vi "sv_Convert Spectrum Info to Variant Attributes.vi"(6 "LabVIEW datatype":T6=3 items=["String: abc"=7, "Boolean: True or False"=8, "Scalar: y"=0, "Array: Y"=1, "Waveform: t0, dt, Y, variant"=2, "Cluster: x0, dx, Y"=3, "Cluster: X, Y"=4, "Waterfall"=5, "Colormap"=6], 8 "error in":errorcluster, 9 "spectrum info":T8 {"x-axis units" items=["Time (s)"=0, "Frequency-CB (Hz)"=1, "Frequency-CPB (Hz)"=1248, "Frequency-Arbitrary (Hz)"=2357, "Quefrency (s)"=2, "Revolutions (rev)"=3, "Order"=4, "Speed (RPM)"=11, "Speed (rad/s)"=21, "Index"=65535]; "weighting filter" items=["Linear", "A-weighting", "B-weighting", "C-weighting", "ITU-R 468-4", "Dolby", "CCITT", "C-message", "Wb", "Wc", "Wd", "We", "Wf", "Wh", "Wj", "Wk", "Wm", "AES17 20 kHz lowpass", "AES17 40 kHz lowpass", "AES17 20 kHz highpass", "AES17 40 kHz highpass"]; "dB reference [EU]" format="%.2f"; "engineering units" items=["custom..."=0, "V"=1, "A"=21, "C"=30, "pC"=31, "s"=32, "-"=29, "Pa"=2, "N"=20, "g"=3, "m/s^2"=4, "m/s"=5, "m"=6, "mm/s"=12, "mm"=13, "micron/s"=14, "micron"=15, "in/s^2"=7, "in/s"=8, "in"=9, "mil/s"=10, "mil"=11, "rad/s^2"=16, "rad/s"=17, "rad"=18, "deg/s^2"=26, "deg/s"=27, "deg"=28, "RPM"=22, "cycle/s^2"=23, "Hz"=24, "cycle"=25, "strain"=19]; "spectral info"."window" items=["None "=0, "Hanning"=1, "Hamming"=2, "Blackman-Harris"=3, "Exact Blackman"=4, "Blackman"=5, "Flat Top"=6, "4 Term B-Harris "=7, "7 Term B-Harris"=8, "Low Sidelobe"=9, "Force - Exponential"=10, "Gaussian"=62]}, 10 "spectrum component":T7 items=["Magnitude"=32, "Phase"=33, "Real"=34, "Imaginary"=35, "Coherence"=36, "Unknown"=99], 11 "attributes in":variant) -> (0 "error out":errorcluster, 1 "unit info":T5, 2 "function info":T4 {"function type" items=["Signal"=0, "Speed"=3, "Ratio"=6, "Count"=7, "-"=9, "Level"=10, "-"=19, "Octave Spectrum"=20, "-"=29, "FFT Auto Spectrum"=30, "FFT Cross Spectrum"=40, "Frequency Response"=50, "-"=59, "Event"=90]; "function subtype" items=["Unscaled binary"=0, "Scaled voltage"=1, "Scaled engineering units"=2, "-"=10, "Value"=19, "DC"=11, "AC"=12, "RMS^2"=13, "RMS"=14, "Peak"=15, "Peak to peak"=16, "-"=20, "1/1 octave"=21, "1/3 octave"=22, "1/6 octave"=23, "1/12 octave"=24, "1/24 octave"=25, "-"=30, "Density"=31, "Magnitude"=32, "Phase"=33, "Real"=34, "Imaginary"=35, "Complex"=345, "Coherence"=36, "-"=90, "Unknown"=99]; "X-domain" items=["Time (s)"=0, "Frequency-CB (Hz)"=1, "Frequency-CPB (Hz)"=1248, "Frequency-Arbitrary (Hz)"=2357, "Quefrency (s)"=2, "Revolutions (rev)"=3, "Order"=4, "Speed (RPM)"=11, "Speed (rad/s)"=21, "Index"=65535]}, 3 "attributes out":variant)   [LabVIEW 2017]
uses:
  <vilib>/addons/_NISVFA/_Shared subVIs/Controls/svc_Spectrum Info.ctl
  <vilib>/addons/_NISVFA/_Shared subVIs/Controls/svc_X-Axis Units.ctl
  <vilib>/addons/_NISVFA/_Shared subVIs/Controls/svc_Spectrum Type.ctl
  <vilib>/addons/_NISVFA/_Shared subVIs/Controls/svc_Engineering Units Text Ring.ctl
  <vilib>/addons/_NISVFA/_Shared subVIs/Controls/svc_Weighting Filter Text Ring.ctl
  <vilib>/addons/_NISVFA/_Shared subVIs/Controls/svc_Complimentary Spectrum Units.ctl
  <vilib>/addons/_NISVFA/_Shared subVIs/Controls/NI Spectrum Component.ctl
  <vilib>/addons/_NISVFA/_Shared subVIs/Controls/LV Datatypes.ctl
  <vilib>/addons/_NISVFA/_Shared subVIs/Controls/NI Function Type.ctl
  <vilib>/addons/_NISVFA/_Shared subVIs/Controls/NI Function SubType.ctl
  <vilib>/addons/_NISVFA/_Shared subVIs/Controls/NI Channel Properties.ctl
  <vilib>/addons/_NISVFA/_Shared subVIs/Controls/SV Channel Properties.ctl
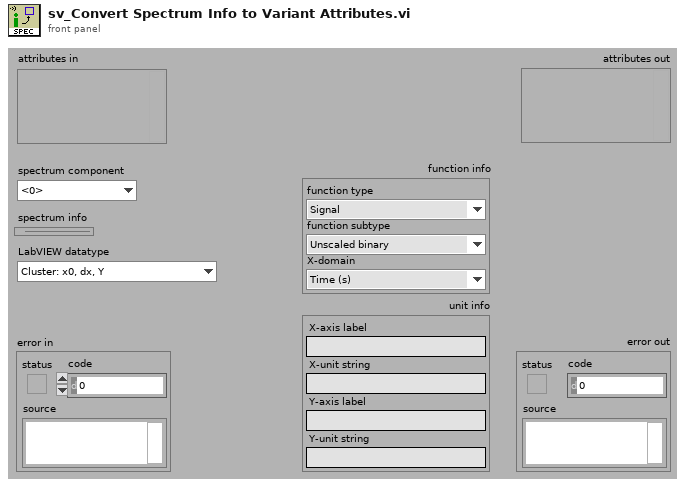
[diagram p1: front panel]
types:
  T1 = typedef "NI Function Type.ctl" = u16
  T2 = typedef "NI Function SubType.ctl" = u16
  T3 = typedef "svc_X-Axis Units.ctl" = u16
  T4 = cluster{"function type":T1, "function subtype":T2, "X-domain":T3}
  T5 = cluster{"X-axis label":string, "X-unit string":string, "Y-axis label":string, "Y-unit string":string}
  T6 = typedef "LV Datatypes.ctl" = i32
  T7 = typedef "NI Spectrum Component.ctl" = u16
  T8 = typedef "svc_Spectrum Info.ctl" = cluster{"channel name":string, "description":string, "x-axis units":T3, "spectral info":cluster{"spectrum type":T9, "linear/dB":enum16{"linear", "dB"}, "window":u16, "window size":i32, "FFT size":i32}, "engineering units":T10, "custom label":string, "dB reference [EU]":dbl, "peak units":enum16{"rms", "peak", "peak-peak"}, "weighting filter":T11, "spectral density?":bool, "unit label":string, "spectrum skewed?":bool, "complimentary spectrum units":T12}
  T9 = typedef "svc_Spectrum Type.ctl" = enum16{"FFT Spectrum [complex]", "Amplitude [Magnitude]", "Power [Magnitude^2]", "Cross Spectrum [complex]", "Frequency Response [Complex]"}
  T10 = typedef "svc_Engineering Units Text Ring.ctl" = u16
  T11 = typedef "svc_Weighting Filter Text Ring.ctl" = u16
  T12 = typedef "svc_Complimentary Spectrum Units.ctl" = enum16{"none", "radians", "degrees", "cycles", "imaginary"}
  T13 = typedef "NI Channel Properties.ctl" = u16
  T14 = typedef "SV Channel Properties.ctl" = u16
  T15 = enum16{"No averaging", "Vector averaging", "RMS averaging", "Peak hold"}
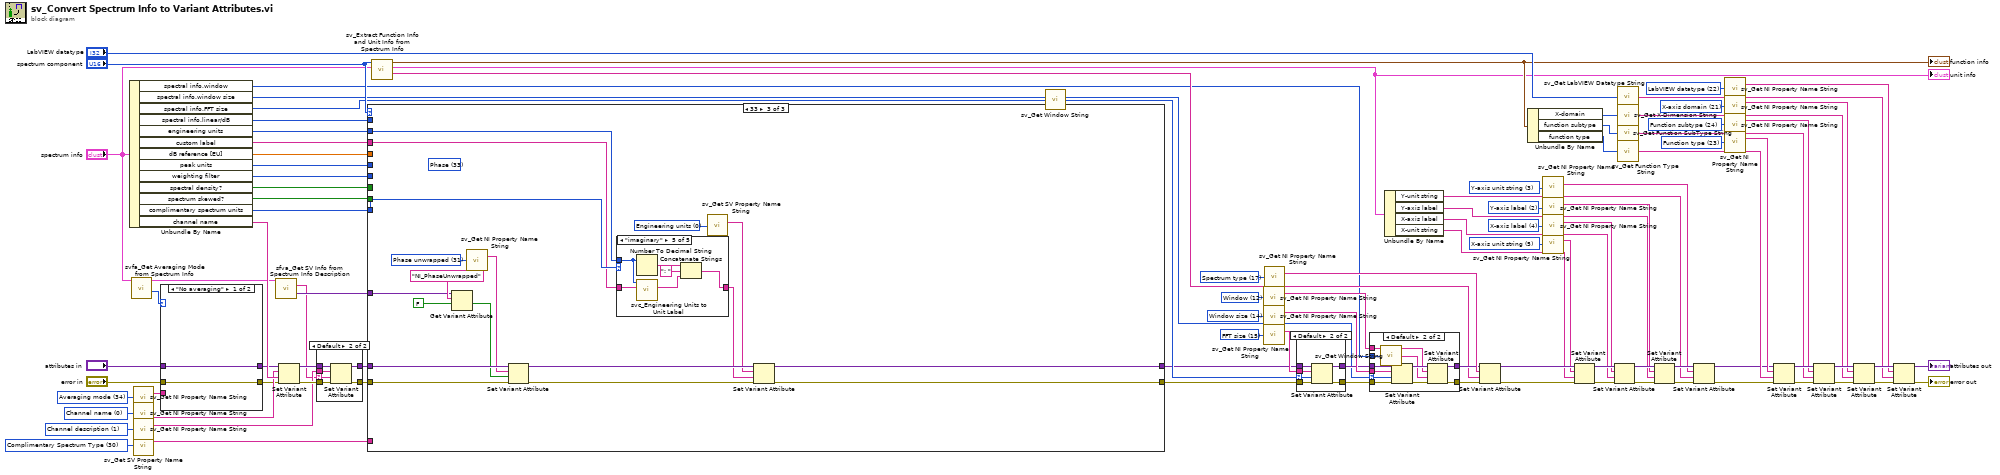
[diagram p0: block diagram]
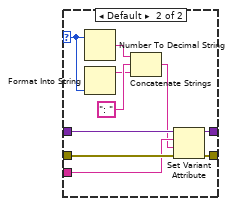
[diagram p2: hidden frame]
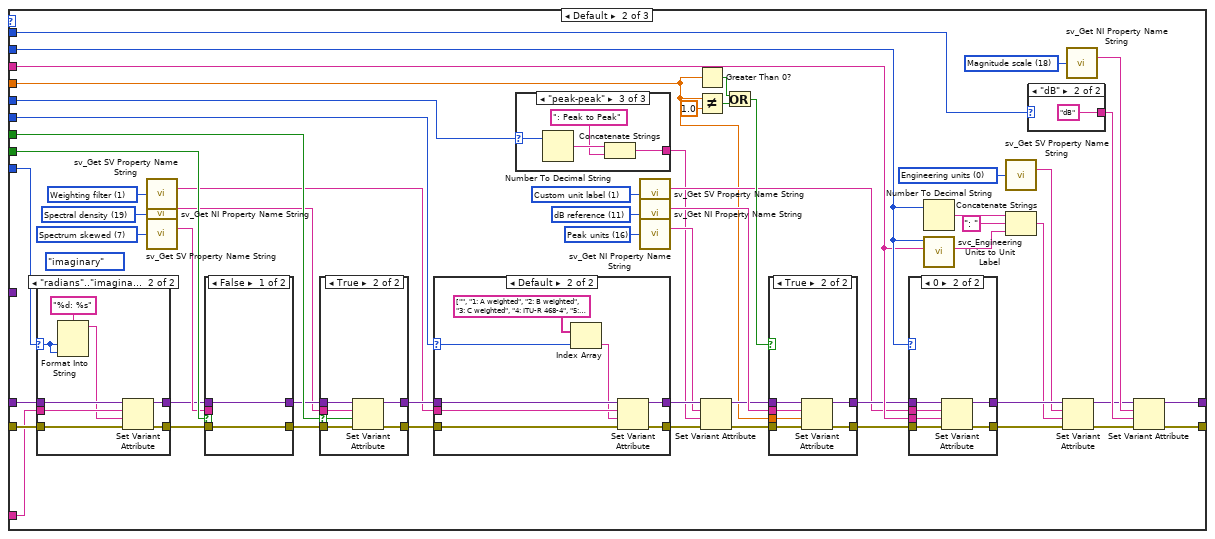
[diagram p7: hidden frame]
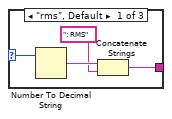
[diagram p10: hidden frame]
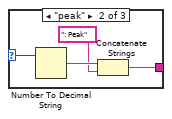
[diagram p11: hidden frame]
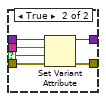
[diagram p12: hidden frame]
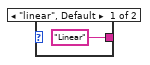
[diagram p13: hidden frame]
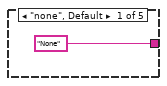
[diagram p17: hidden frame]
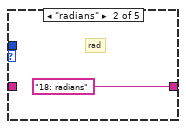
[diagram p18: hidden frame]
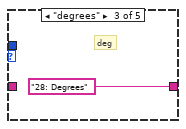
[diagram p19: hidden frame]
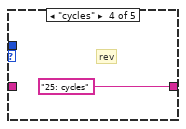
[diagram p20: hidden frame]
diagram:
  w3 = T13 34 items=["Channel name", "Channel description", "Axis label", "Unit string", "Waveform X-axis label", "Waveform X-axis unit string", "x0", "dx", "Number of samples", "X channel", "Filter settled", "dB reference", "Window", "Window parameter", "Window size", "FFT size", "Peak units", "Spectrum type", "Magnitude scale", "Spectral density", "Sensor sensitivity (mV/EU)", "X-axis dimension", "LabVIEW datatype", "Function type", "Function subtype", "X values", "Independent channel", "Column index", "Collection name", "Collection ID", "X Columns", "Phase unwrapped", "Sensor type", "Sensor maximum", "Averaging mode"] ("property")
  w12 = T14 30 items=["Engineering units", "Custom unit label", "Weighting filter", "Pregain", "Octave standard", "Octave bandwidth", "Octave low band", "Octave high band", "Spectrum skewed", "Samples / revolution", "Order", "Tachometer", "Pulses Per Revolution", "Rotation Direction", "Probe Angle", "Pair", "Channel Alias", "Tachometer Threshold", "Tachometer Slope", "Max Order", "Sensor Location", "Sensor Orientation", "Analog Software Trigger", "Trigger Level", "Pretrigger Samples", "Trigger Slope", "Trigger Hysteresis", "Sensor sensitivity", "Sensor type", "Sensor maximum", "Complimentary Spectrum Type"] ("property")
  w33 = T13 2 items=["Channel name", "Channel description", "Y-axis label", "Y-axis unit string", "X-axis label", "X-axis unit string", "x0", "dx", "Number of samples", "X channel", "Filter settled", "dB reference", "Window", "Window parameter", "Window size", "FFT size", "Peak units", "Spectrum type", "Magnitude scale", "Spectral density", "Sensor sensitivity (mV/EU)", "X-axis domain", "LabVIEW datatype"] ("property")
  w32 = T13 3 items=["Channel name", "Channel description", "Y-axis label", "Y-axis unit string", "X-axis label", "X-axis unit string", "x0", "dx", "Number of samples", "X channel", "Filter settled", "dB reference", "Window", "Window parameter", "Window size", "FFT size", "Peak units", "Spectrum type", "Magnitude scale", "Spectral density", "Sensor sensitivity (mV/EU)", "X-axis domain", "LabVIEW datatype"] ("property")
  w35 = T13 5 items=["Channel name", "Channel description", "Y-axis label", "Y-axis unit string", "X-axis label", "X-axis unit string", "x0", "dx", "Number of samples", "X channel", "Filter settled", "dB reference", "Window", "Window parameter", "Window size", "FFT size", "Peak units", "Spectrum type", "Magnitude scale", "Spectral density", "Sensor sensitivity (mV/EU)", "X-axis domain", "LabVIEW datatype"] ("property")
  w36 = T13 4 items=["Channel name", "Channel description", "Y-axis label", "Y-axis unit string", "X-axis label", "X-axis unit string", "x0", "dx", "Number of samples", "X channel", "Filter settled", "dB reference", "Window", "Window parameter", "Window size", "FFT size", "Peak units", "Spectrum type", "Magnitude scale", "Spectral density", "Sensor sensitivity (mV/EU)", "X-axis domain", "LabVIEW datatype"] ("property")
  w49 = T13 15 items=["Channel name", "Channel description", "Y-axis label", "Y-axis unit string", "X-axis label", "X-axis unit string", "x0", "dx", "Number of samples", "X channel", "Filter settled", "dB reference", "Window", "Window parameter", "Window size", "FFT size", "Peak units", "Spectrum type", "Magnitude scale", "Spectral density"] ("property")
  w48 = T13 14 items=["Channel name", "Channel description", "Y-axis label", "Y-axis unit string", "X-axis label", "X-axis unit string", "x0", "dx", "Number of samples", "X channel", "Filter settled", "dB reference", "Window", "Window parameter", "Window size", "FFT size", "Peak units", "Spectrum type", "Magnitude scale", "Spectral density"] ("property")
  w45 = T13 12 items=["Channel name", "Channel description", "Y-axis label", "Y-axis unit string", "X-axis label", "X-axis unit string", "x0", "dx", "Number of samples", "X channel", "Filter settled", "dB reference", "Window", "Window parameter", "Window size", "FFT size", "Peak units", "Spectrum type", "Magnitude scale", "Spectral density"] ("property")
  w70 = T13 22 items=["Channel name", "Channel description", "Y-axis label", "Y-axis unit string", "X-axis label", "X-axis unit string", "x0", "dx", "Number of samples", "X channel", "Filter settled", "dB reference", "Window", "Window parameter", "Window size", "FFT size", "Peak units", "Spectrum type", "Magnitude scale", "Spectral density", "Sensor sensitivity (mV/EU)", "X-axis domain", "LabVIEW datatype"] ("property")
  w73 = T13 24 items=["Channel name", "Channel description", "Y-axis label", "Y-axis unit string", "X-axis label", "X-axis unit string", "x0", "dx", "Number of samples", "X channel", "Filter settled", "dB reference", "Window", "Window parameter", "Window size", "FFT size", "Peak units", "Spectrum type", "Magnitude scale", "Spectral density", "Sensor sensitivity (mV/EU)", "X-axis dimension", "LabVIEW datatype", "Function type", "Function subtype"] ("property")
  w74 = T13 21 items=["Channel name", "Channel description", "Y-axis label", "Y-axis unit string", "X-axis label", "X-axis unit string", "x0", "dx", "Number of samples", "X channel", "Filter settled", "dB reference", "Window", "Window parameter", "Window size", "FFT size", "Peak units", "Spectrum type", "Magnitude scale", "Spectral density", "Sensor sensitivity (mV/EU)", "X-axis domain", "LabVIEW datatype", "Function type", "Component", "Level detector"] ("property")
  w72 = T13 23 items=["Channel name", "Channel description", "Y-axis label", "Y-axis unit string", "X-axis label", "X-axis unit string", "x0", "dx", "Number of samples", "X channel", "Filter settled", "dB reference", "Window", "Window parameter", "Window size", "FFT size", "Peak units", "Spectrum type", "Magnitude scale", "Spectral density", "Sensor sensitivity (mV/EU)", "X-axis domain", "LabVIEW datatype", "Function type", "Component", "Level detector"] ("property")
  w93 = T13 17 items=["Channel name", "Channel description", "Y-axis label", "Y-axis unit string", "X-axis label", "X-axis unit string", "x0", "dx", "Number of samples", "X channel", "Filter settled", "dB reference", "Window", "Window parameter", "Window size", "FFT size", "Peak units", "Spectrum type", "Magnitude scale", "Spectral density"] ("property")
  w92 = T13 0 items=["Channel name", "Channel description", "Y-axis label", "Y-axis unit string", "X-axis label", "X-axis unit string", "x0", "dx", "Number of samples", "X channel", "Filter settled", "dB reference", "Window", "Window parameter", "Window size", "FFT size", "Peak units", "Spectrum type", "Magnitude scale", "Spectral density"] ("property")
  w91 = T13 1 items=["Channel name", "Channel description", "Y-axis label", "Y-axis unit string", "X-axis label", "X-axis unit string", "x0", "dx", "Number of samples", "X channel", "Filter settled", "dB reference", "Window", "Window parameter", "Window size", "FFT size", "Peak units", "Spectrum type", "Magnitude scale", "Spectral density"] ("property")
  n1 = Unbundle By Name("spectrum info") -> ("spectral info.window"=w13:u16, "spectral info.window size"=w39:i32, "spectral info.FFT size"=w44:i32, "spectral info.linear/dB"=w84:enum16{"linear", "dB"}, "engineering units"=w85:T10, "custom label"=w86:string, "dB reference [EU]"=w87:dbl, "peak units"=w90:enum16{"rms", "peak", "peak-peak"}, "weighting filter"=w88:T11, "spectral density?"=w95:bool, "spectrum skewed?"=w83:bool, "complimentary spectrum units"=w89:T12, "channel name"=w37:string)
  n2 = call <vilib>:"svfa_Get Averaging Mode from Spectrum Info.vi"("spectrum info"="spectrum info") -> ("averaging mode"=w1:T15, "spectrum info"=w8:T8)  [unwired: 8 in, 1 out]
  n3 = call <vilib>:"sv_Get NI Property Name String.vi"("property"=w3) -> ("TDMS property name"=w2:string)  [unwired: 13 in, 1 out]
  n4 = call <vilib>:"sv_Get NI Property Name String.vi"("property"=w92) -> ("WDT attribute name"=w10:string)  [unwired: 13 in, 1 out]
  n5 = call <vilib>:"sv_Get NI Property Name String.vi"("property"=w91) -> ("TDMS property name"=w80:string)  [unwired: 13 in, 1 out]
  n6 = call <vilib>:"sv_Get SV Property Name String.vi"("property"=w12) -> ("TDMS property name"=w11:string)  [unwired: 13 in, 1 out]
  n7 = case shown="\"No averaging\"" w1 {
    selector: w1 -> [_ w102]
    tunnel: "attributes in" -> [w100 w110]
    tunnel: [w100 w109] -> w6
    tunnel: "error in" -> [w99 w108]
    tunnel: [w99 w107] -> w4
    tunnel: w2 -> [_ w106]
    frame "No averaging" {
    }
    frame Default {
      n8 = Number To Decimal String(number=w102) -> (decimal integer string=w104:string)  [unwired: 1 in]
      n9 = Format Into String(w102) -> (resulting string=w103:string)  [unwired: 3 in, 1 out]
      n10 = Concatenate Strings(w104, ": " ("string"), w103) -> (w101:string)
      n11 = Set Variant Attribute(Variant=w110, name=w106, value=w101, error in=w108) -> (Variant out=w109:variant, error out=w107:errorcluster)  [unwired: 1 out]
    }
  }
  n12 = call <vilib>:"sfva_Get SV Info from Spectrum Info Description.vi"("spectrum info"=w8) -> ("description"=w79:string, "SV Info"=w98:variant)  [unwired: 10 in, 3 out]
  n13 = Set Variant Attribute(Variant=w6, name=w10, value=w37, error in=w4) -> (Variant out=w82:variant, error out=w81:errorcluster)  [unwired: 1 out]
  n14 = case shown="Default" w79 {
    selector: w79 -> [_ w114]
    tunnel: [w112 w115] -> w96
    tunnel: [w111 w117] -> w97
    tunnel: w81 -> [w111 w118]
    tunnel: w82 -> [w112 w116]
    tunnel: w80 -> [_ w113]
    frame "" {
    }
    frame Default {
      n15 = Set Variant Attribute(Variant=w116, name=w113, value=w114, error in=w118) -> (Variant out=w115:variant, error out=w117:errorcluster)  [unwired: 1 out]
    }
  }
  n16 = case shown="33" "spectrum component" {
    tunnel: w83 -> [_ w167 _]
    tunnel: w84 -> [_ w176 _]
    tunnel: [w120 w130 w243] -> w43
    tunnel: [w119 w139 w256] -> w42
    tunnel: w96 -> [w120 w126 w253]
    tunnel: w97 -> [w119 w124 w252]
    tunnel: w85 -> [_ w165 w259]
    tunnel: w86 -> [_ w164 w258]
    tunnel: w87 -> [_ w127 _]
    tunnel: w88 -> [_ w166 _]
    tunnel: w95 -> [_ w169 _]
    tunnel: w89 -> [_ w122 w260]
    tunnel: w90 -> [_ w168 _]
    tunnel: w98 -> [_ _ w254]
    tunnel: w11 -> [_ w121 _]
    frame 36 {
    }
    frame Default {
      (unwired) svc_Complimentary_Spectrum_Units."imaginary" ("complimentary spectrum units")
      w140 = T14 0 items=["Engineering units", "Weighting filter", "Pregain", "Octave standard", "Octave bandwidth", "Octave low band", "Octave high band", "Spectrum skewed"] ("property")
      w141 = T13 18 items=["Channel name", "Channel description", "Y-axis label", "Y-axis unit string", "X-axis label", "X-axis unit string", "x0", "dx", "Number of samples", "X channel", "Filter settled", "dB reference", "Window", "Window parameter", "Window size", "FFT size", "Peak units", "Spectrum type", "Magnitude scale", "Spectral density"] ("property")
      w144 = T14 1 items=["Engineering units", "Custom unit label", "Weighting filter", "Pregain", "Octave standard", "Octave bandwidth", "Octave low band", "Octave high band", "Spectrum skewed"] ("property")
      w145 = T13 11 items=["Channel name", "Channel description", "Y-axis label", "Y-axis unit string", "X-axis label", "X-axis unit string", "x0", "dx", "Number of samples", "X channel", "Filter settled", "dB reference", "Window", "Window parameter", "Window size", "FFT size", "Peak units", "Spectrum type", "Magnitude scale", "Spectral density"] ("property")
      w146 = T13 16 items=["Channel name", "Channel description", "Y-axis label", "Y-axis unit string", "X-axis label", "X-axis unit string", "x0", "dx", "Number of samples", "X channel", "Filter settled", "dB reference", "Window", "Window parameter", "Window size", "FFT size", "Peak units", "Spectrum type", "Magnitude scale", "Spectral density"] ("property")
      w148 = T13 19 items=["Channel name", "Channel description", "Y-axis label", "Y-axis unit string", "X-axis label", "X-axis unit string", "x0", "dx", "Number of samples", "X channel", "Filter settled", "dB reference", "Window", "Window parameter", "Window size", "FFT size", "Peak units", "Spectrum type", "Magnitude scale", "Spectral density"] ("property")
      w149 = T14 7 items=["Engineering units", "Weighting filter", "Pregain", "Octave standard", "Octave bandwidth", "Octave low band", "Octave high band", "Spectrum skewed"] ("property")
      w150 = T14 1 items=["Engineering units", "Weighting filter", "Pregain", "Octave standard", "Octave bandwidth", "Octave low band", "Octave high band", "Spectrum skewed"] ("property")
      n17 = case shown="\"radians\"..\"imaginary\"" w122 {
        selector: w122 -> [_ w180]
        tunnel: w126 -> [w178 w186]
        tunnel: [w178 w185] -> w125
        tunnel: w124 -> [w177 w184]
        tunnel: [w177 w183] -> w123
        tunnel: w121 -> [_ w182]
        frame "none", Default {
        }
        frame "radians".."imaginary" {
          n18 = Format Into String(format string="%d: %s", w180, w180) -> (resulting string=w179:string)  [unwired: 2 in, 1 out]
          n19 = Set Variant Attribute(Variant=w186, name=w182, value=w179, error in=w184) -> (Variant out=w185:variant, error out=w183:errorcluster)  [unwired: 1 out]
        }
      }
      n20 = call <vilib>:"sv_Get SV Property Name String.vi"("property"=w150) -> ("TDMS property name"=w151:string)  [unwired: 13 in, 1 out]
      n21 = call <vilib>:"sv_Get NI Property Name String.vi"("property"=w148) -> ("TDMS property name"=w147:string)  [unwired: 13 in, 1 out]
      n22 = call <vilib>:"sv_Get SV Property Name String.vi"("property"=w149) -> ("TDMS property name"=w138:string)  [unwired: 13 in, 1 out]
      n23 = case shown="False" w167 {
        selector: w167 -> [_ w213]
        tunnel: w123 -> [w207 w212]
        tunnel: w125 -> [w208 w211]
        tunnel: [w208 w209] -> w153
        tunnel: [w207 w210] -> w152
        tunnel: w138 -> [_ w214]
        frame False {
        }
        frame True {
          n24 = Set Variant Attribute(Variant=w211, name=w214, value=w213, error in=w212) -> (Variant out=w209:variant, error out=w210:errorcluster)  [unwired: 1 out]
        }
      }
      n25 = case shown="True" w169 {
        selector: w169 -> [_ w237]
        tunnel: w152 -> [w235 w242]
        tunnel: w153 -> [w236 w241]
        tunnel: [w236 w239] -> w170
        tunnel: [w235 w240] -> w171
        tunnel: w147 -> [_ w238]
        frame False {
        }
        frame True {
          n26 = Set Variant Attribute(Variant=w241, name=w238, value=w237, error in=w242) -> (Variant out=w239:variant, error out=w240:errorcluster)  [unwired: 1 out]
        }
      }
      n27 = case shown="Default" w166 {
        selector: w166 -> [_ w231]
        tunnel: w171 -> [w225 w234]
        tunnel: w170 -> [w226 w233]
        tunnel: [w226 w227] -> w173
        tunnel: [w225 w232] -> w172
        tunnel: w151 -> [_ w229]
        frame 0 {
        }
        frame Default {
          n28 = Index Array(array=string[] ["", "1: A weighted", "2: B weighted", "3: C weighted", "4: ITU-R 468-4", "5: Dolby", "6: CCITT", "7: C-message", "8: Wb", "9: Wc", "10: Wd", "11: We", "12: Wf", "13: Wh", "14: Wj", "15: Wk", "16: Wm"] ("transposed array"), index=w231) -> (element=w228:string)
          n29 = Set Variant Attribute(Variant=w233, name=w229, value=w228, error in=w234) -> (Variant out=w227:variant, error out=w232:errorcluster)  [unwired: 1 out]
        }
      }
      n30 = case shown="\"peak-peak\"" w168 {
        selector: w168 -> [w198 w202 w206]
        tunnel: [w196 w200 w204] -> w136
        frame "rms", Default {
          n31 = Number To Decimal String(number=w198) -> (decimal integer string=w197:string)  [unwired: 1 in]
          n32 = Concatenate Strings(w197, ": RMS" ("string")) -> (w196:string)
        }
        frame "peak" {
          n33 = Number To Decimal String(number=w202) -> (decimal integer string=w201:string)  [unwired: 1 in]
          n34 = Concatenate Strings(w201, ": Peak" ("string")) -> (w200:string)
        }
        frame "peak-peak" {
          n35 = Number To Decimal String(number=w206) -> (decimal integer string=w205:string)  [unwired: 1 in]
          n36 = Concatenate Strings(w205, ": Peak to Peak" ("string")) -> (w204:string)
        }
      }
      n37 = call <vilib>:"sv_Get SV Property Name String.vi"("property"=w144) -> ("TDMS property name"=w143:string)  [unwired: 13 in, 1 out]
      n38 = call <vilib>:"sv_Get NI Property Name String.vi"("property"=w145) -> ("TDMS property name"=w142:string)  [unwired: 13 in, 1 out]
      n39 = call <vilib>:"sv_Get NI Property Name String.vi"("property"=w146) -> ("TDMS property name"=w137:string)  [unwired: 13 in, 1 out]
      n40 = Greater Than 0?(x=w127) -> (x > 0?=w157:bool)
      n41 = Not Equal?(x=w127, y=1.0 ("x")) -> (x != y?=w158:bool)
      n42 = Set Variant Attribute(Variant=w173, name=w137, value=w136, error in=w172) -> (Variant out=w135:variant, error out=w162:errorcluster)  [unwired: 1 out]
      n43 = Or(x=w157, y=w158) -> (x .or. y?=w156:bool)
      n44 = case shown="True" w156 {
        tunnel: w162 -> [w188 w194]
        tunnel: [w187 w189] -> w161
        tunnel: [w188 w193] -> w160
        tunnel: w142 -> [_ w190]
        tunnel: w127 -> [_ w191]
        tunnel: w135 -> [w187 w192]
        frame False {
        }
        frame True {
          n45 = Set Variant Attribute(Variant=w192, name=w190, value=w191, error in=w194) -> (Variant out=w189:variant, error out=w193:errorcluster)  [unwired: 1 out]
        }
      }
      n46 = case shown="0" w165 {
        tunnel: w160 -> [w217 w224]
        tunnel: w161 -> [w218 w223]
        tunnel: [w218 w219] -> w175
        tunnel: [w217 w222] -> w174
        tunnel: w143 -> [_ w221]
        tunnel: w164 -> [_ w220]
        frame Default {
        }
        frame 0 {
          n47 = Set Variant Attribute(Variant=w223, name=w221, value=w220, error in=w224) -> (Variant out=w219:variant, error out=w222:errorcluster)  [unwired: 1 out]
        }
      }
      n48 = Number To Decimal String(number=w165) -> (decimal integer string=w155:string)  [unwired: 1 in]
      n49 = call <vilib>:"svc_Engineering Units to Unit Label.vi"("custom label"=w164, "engineering units"=w165) -> ("unit label"=w154:string)  [unwired: 8 in, 1 out]
      n50 = call <vilib>:"sv_Get SV Property Name String.vi"("property"=w140) -> ("TDMS property name"=w133:string)  [unwired: 13 in, 1 out]
      n51 = Concatenate Strings(w155, ": " ("string"), w154) -> (w134:string)
      n52 = case shown="\"dB\"" w176 {
        tunnel: ["Linear" ("t") "dB" ("f")] -> w131
        frame "linear", Default {
        }
        frame "dB" {
        }
      }
      n53 = Set Variant Attribute(Variant=w175, name=w133, value=w134, error in=w174) -> (Variant out=w129:variant, error out=w128:errorcluster)  [unwired: 1 out]
      n54 = call <vilib>:"sv_Get NI Property Name String.vi"("property"=w141) -> ("TDMS property name"=w132:string)  [unwired: 13 in, 1 out]
      n55 = Set Variant Attribute(Variant=w129, name=w132, value=w131, error in=w128) -> (Variant out=w130:variant, error out=w139:errorcluster)  [unwired: 1 out]
    }
    frame 33 {
      (unwired) T7 33 items=["Magnitude"=32, "Phase"=33, "Real"=34, "Imaginary"=35, "Coherence"=36, "Unknown"=99] ("spectrum component")
      w250 = T13 31 items=["Channel name", "Channel description", "Axis label", "Unit string", "Waveform X-axis label", "Waveform X-axis unit string", "x0", "dx", "Number of samples", "X channel", "Filter settled", "dB reference", "Window", "Window parameter", "Window size", "FFT size", "Peak units", "Spectrum type", "Magnitude scale", "Spectral density", "Sensor sensitivity (mV/EU)", "X-axis dimension", "LabVIEW datatype", "Function type", "Function subtype", "X values", "Independent channel", "Column index", "Collection name", "Collection ID", "X Columns", "Phase unwrapped"] ("property")
      w257 = T14 0 items=["Engineering units", "Custom unit label", "Weighting filter", "Pregain", "Octave standard", "Octave bandwidth", "Octave low band", "Octave high band", "Spectrum skewed"] ("SV property")
      n56 = Get Variant Attribute(Variant=w254, name="NI_PhaseUnwrapped", default value (empty Variant)=FALSE ("unwrap phase? (T)")) -> (value=w247:bool)  [unwired: 1 in, 3 out]
      n57 = call <vilib>:"sv_Get NI Property Name String.vi"("property"=w250) -> ("TDMS property name"=w248:string)  [unwired: 13 in, 1 out]
      n58 = Set Variant Attribute(Variant=w253, name=w248, value=w247, error in=w252) -> (Variant out=w246:variant, error out=w251:errorcluster)  [unwired: 1 out]
      n59 = case shown="\"imaginary\"" w260 {
        tunnel: ["None" ("string") "18: radians" ("string") "28: Degrees" ("string") "25: cycles" ("string") w265] -> w244
        tunnel: w259 -> [_ _ _ _ w267]
        tunnel: w258 -> [_ _ _ _ w266]
        frame "none", Default {
        }
        frame "radians" {
          # "rad"
        }
        frame "degrees" {
          # "deg"
        }
        frame "cycles" {
          # "rev"
        }
        frame "imaginary" {
          n60 = Number To Decimal String(number=w267) -> (decimal integer string=w269:string)  [unwired: 1 in]
          n61 = call <vilib>:"svc_Engineering Units to Unit Label.vi"("custom label"=w266, "engineering units"=w267) -> ("unit label"=w268:string)  [unwired: 8 in, 1 out]
          n62 = Concatenate Strings(w269, ": " ("string"), w268) -> (w265:string)
        }
      }
      n63 = call <vilib>:"sv_Get SV Property Name String.vi"("property"=w257) -> ("TDMS property name"=w245:string)  [unwired: 13 in, 1 out]
      n64 = Set Variant Attribute(Variant=w246, name=w245, value=w244, error in=w251) -> (Variant out=w243:variant, error out=w256:errorcluster)  [unwired: 1 out]
      n65 = call <vilib>:"sv_Get Window String.vi"() -> ()  [unwired: 5 in, 1 out]
    }
  }
  n66 = call <vilib>:"sv_Extract Function Info and Unit Info from Spectrum Info.vi"("spectrum info"="spectrum info", "spectrum component"="spectrum component") -> ("spectrum info.spectrum type string"=w38:string, "unit info"=w34:T5, "function info"=w55:T4)  [unwired: 7 in]
  "unit info" <- w34
  "function info" <- w55
  n67 = call <vilib>:"sv_Get NI Property Name String.vi"("property"=w45) -> ("TDMS property name"=w52:string)  [unwired: 13 in, 1 out]
  n68 = call <vilib>:"sv_Get NI Property Name String.vi"("property"=w48) -> ("TDMS property name"=w51:string)  [unwired: 13 in, 1 out]
  n69 = call <vilib>:"sv_Get NI Property Name String.vi"("property"=w49) -> ("TDMS property name"=w50:string)  [unwired: 13 in, 1 out]
  n70 = call <vilib>:"sv_Get NI Property Name String.vi"("property"=w93) -> ("TDMS property name"=w78:string)  [unwired: 13 in, 1 out]
  n71 = case shown="Default" w44 {
    selector: w44 -> [_ w275]
    tunnel: w50 -> [_ w276]
    tunnel: [w272 w277] -> w46
    tunnel: [w271 w278] -> w47
    tunnel: w43 -> [w272 w274]
    tunnel: w42 -> [w271 w273]
    frame 0 {
    }
    frame Default {
      n72 = Set Variant Attribute(Variant=w274, name=w276, value=w275, error in=w273) -> (Variant out=w277:variant, error out=w278:errorcluster)  [unwired: 1 out]
    }
  }
  n73 = case shown="Default" w39 {
    selector: w39 -> [_ w284]
    tunnel: w52 -> [_ w283]
    tunnel: w51 -> [_ w285]
    tunnel: [w279 w291] -> w40
    tunnel: [w280 w286] -> w41
    tunnel: w46 -> [w280 w289]
    tunnel: w47 -> [w279 w288]
    tunnel: w13 -> [_ w281]
    frame 0 {
    }
    frame Default {
      n74 = call <vilib>:"sv_Get Window String.vi"("window"=w281) -> ("window string"=w282:string)  [unwired: 4 in]
      n75 = Set Variant Attribute(Variant=w289, name=w285, value=w284, error in=w288) -> (Variant out=w287:variant, error out=w290:errorcluster)  [unwired: 1 out]
      n76 = Set Variant Attribute(Variant=w287, name=w283, value=w282, error in=w290) -> (Variant out=w286:variant, error out=w291:errorcluster)  [unwired: 1 out]
    }
  }
  n77 = Unbundle By Name(w34) -> ("Y-unit string"=w21:string, "Y-axis label"=w18:string, "X-axis label"=w17:string, "X-unit string"=w15:string)
  n78 = Set Variant Attribute(Variant=w41, name=w78, value=w38, error in=w40) -> (Variant out=w25:variant, error out=w24:errorcluster)  [unwired: 1 out]
  n79 = Unbundle By Name(w55) -> ("X-domain"=w76:T3, "function subtype"=w75:T2, "function type"=w77:T1)
  n80 = call <vilib>:"sv_Get NI Property Name String.vi"("property"=w32) -> ("TDMS property name"=w20:string)  [unwired: 13 in, 1 out]
  n81 = call <vilib>:"sv_Get NI Property Name String.vi"("property"=w33) -> ("TDMS property name"=w19:string)  [unwired: 13 in, 1 out]
  n82 = call <vilib>:"sv_Get NI Property Name String.vi"("property"=w36) -> ("TDMS property name"=w16:string)  [unwired: 13 in, 1 out]
  n83 = call <vilib>:"sv_Get NI Property Name String.vi"("property"=w35) -> ("TDMS property name"=w14:string)  [unwired: 13 in, 1 out]
  n84 = Set Variant Attribute(Variant=w25, name=w14, value=w15, error in=w24) -> (Variant out=w31:variant, error out=w30:errorcluster)  [unwired: 1 out]
  n85 = Set Variant Attribute(Variant=w31, name=w16, value=w17, error in=w30) -> (Variant out=w29:variant, error out=w28:errorcluster)  [unwired: 1 out]
  n86 = call <vilib>:"sv_Get LabVIEW Datatype String.vi"("LabVIEW datatype"="LabVIEW datatype") -> ("datatype string"=w56:string)  [unwired: 4 in]
  n87 = call <vilib>:"sv_Get X-Dimension String.vi"("x-axis units"=w76) -> ("x-domain string"=w58:string)  [unwired: 4 in]
  n88 = call <vilib>:"sv_Get Function SubType String.vi"("function subtype"=w75) -> ("function type string"=w60:string)  [unwired: 4 in]
  n89 = call <vilib>:"sv_Get Function Type String.vi"("function type"=w77) -> ("function type string"=w62:string)  [unwired: 4 in]
  n90 = Set Variant Attribute(Variant=w29, name=w19, value=w18, error in=w28) -> (Variant out=w27:variant, error out=w26:errorcluster)  [unwired: 1 out]
  n91 = Set Variant Attribute(Variant=w27, name=w20, value=w21, error in=w26) -> (Variant out=w23:variant, error out=w22:errorcluster)  [unwired: 1 out]
  n92 = call <vilib>:"sv_Get NI Property Name String.vi"("property"=w70) -> ("TDMS property name"=w57:string)  [unwired: 13 in, 1 out]
  n93 = call <vilib>:"sv_Get NI Property Name String.vi"("property"=w74) -> ("TDMS property name"=w59:string)  [unwired: 13 in, 1 out]
  n94 = call <vilib>:"sv_Get NI Property Name String.vi"("property"=w73) -> ("TDMS property name"=w61:string)  [unwired: 13 in, 1 out]
  n95 = call <vilib>:"sv_Get NI Property Name String.vi"("property"=w72) -> ("TDMS property name"=w63:string)  [unwired: 13 in, 1 out]
  n96 = Set Variant Attribute(Variant=w23, name=w63, value=w62, error in=w22) -> (Variant out=w64:variant, error out=w65:errorcluster)  [unwired: 1 out]
  n97 = Set Variant Attribute(Variant=w64, name=w61, value=w60, error in=w65) -> (Variant out=w66:variant, error out=w67:errorcluster)  [unwired: 1 out]
  n98 = Set Variant Attribute(Variant=w66, name=w59, value=w58, error in=w67) -> (Variant out=w68:variant, error out=w69:errorcluster)  [unwired: 1 out]
  n99 = Set Variant Attribute(Variant=w68, name=w57, value=w56, error in=w69) -> (Variant out=→"attributes out":variant, error out=→"error out":errorcluster)  [unwired: 1 out]
